vi "RVHR - Get Sum File Info.vi"(6 "Local Data in":T1, 8 "error in (no error)":errorcluster, 11 ".sum filepath":path) -> (0 "error out":errorcluster, 4 "Local Data out":T1)   [LabVIEW 2024]
uses:
  Controls/RVHR - Local Data.ctl
  Controls/Test Cluster.ctl
  Controls/Excluded Information.ctl
  Controls/Language.ctl
  Controls/Device_Type.ctl
  <vilib>/Utility/miscctls.llb/LVRectTypeDef.ctl
  <vilib>/Utility/miscctls.llb/LVBoundsTypeDef.ctl
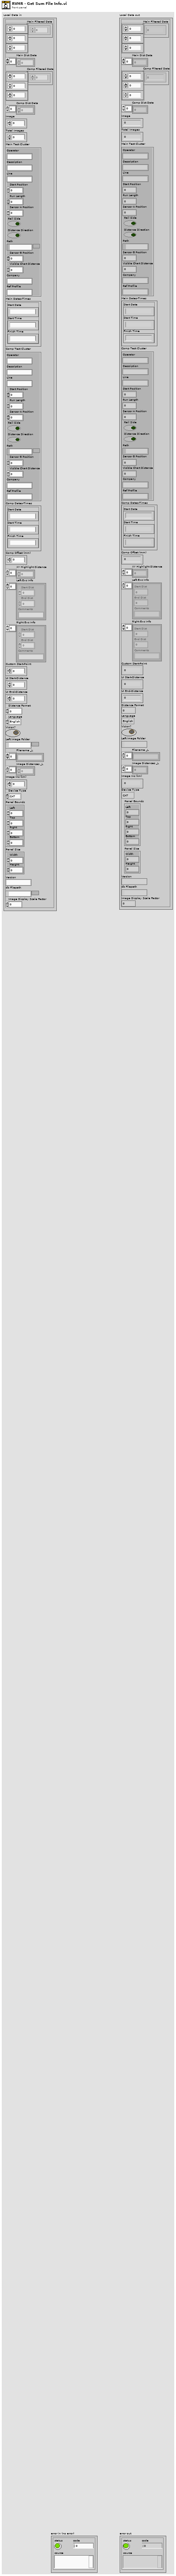
[diagram p1: front panel]
types:
  T1 = typedef "RVHR - Local Data.ctl" = cluster{"Main Filtered Data":dbl[][][], "Main Dist Data":dbl[], "Comp Filtered Data":dbl[][][], "Comp Dist Data":dbl[], "Image":u16, "Total Images":u16, "Main Test Cluster":T2, "Main Dates-Times":cluster{"Start Date":string, "Start Time":string, "Finish Time":string}, "Comp Test Cluster":T2, "Comp Dates-Times":cluster{"Start Date":string, "Start Time":string, "Finish Time":string}, "Comp Offset (mm)":i64, "XY Highlight Distance":dbl[], "Left Exc Info":T3[], "Right Exc Info":T3[], "Custom Start-Point":dbl, "UI Start-Distance":dbl, "UI End-Distance":dbl, "Distance Format":u8, "Language":T4, "Vision?":bool, "Left Image Folder":path, "Filename _L":string[], "Image Distances _L":dbl[], "Image Inc (km)":dbl, "Device Type":T5, "Panel Bounds":T6, "Panel Size":T7, "Version":string, "db Filepath":path, "Image Display Scale Factor":dbl}
  T2 = typedef "Test Cluster.ctl" = cluster{"Operator":string, "Description":string, "Line":string, "Start Position":dbl, "Run Length":dbl, "Sensor A Position":dbl, "Rail Side":bool, "Distance Direction":bool, "Path":path, "Sensor B Position":dbl, "Visible Chart Distance":dbl, "Company":string, "Ref Profile":string}
  T3 = typedef "Excluded Information.ctl" = cluster{"Start Dist":dbl, "End Dist":dbl, "Comments":string}
  T4 = typedef "Language.ctl" = enum16{"English", "Chinese", "German"}
  T5 = typedef "Device_Type.ctl" = enum16{"CAT", "Bi-CAT", "YRCA", "RCA", "RV-HR", "TV-HR"}
  T6 = typedef "LVRectTypeDef.ctl" = cluster{"Left":i16, "Top":i16, "Right":i16, "Bottom":i16}
  T7 = typedef "LVBoundsTypeDef.ctl" = cluster{"Width":u32, "Height":u32}
  T8 = cluster{"Start Date":string, "Start Time":string, "Finish Time":string}
  T9 = typedef "SUM Cluster.ctl" = cluster{"Test Cluster":T2, "Settings Cluster":T10, "End Distance":dbl, "Current Pos":dbl, "Start Pos":dbl, "Device_Type":T5, "Version":string}
  T10 = typedef "Settings Cluster.ctl" = cluster{"Sensor A Calibration":dbl, "Integrator Time":dbl, "Encoder Spacing":dbl, "Encoder Threshold":dbl, "Sampling Distance":T11, "Swap Direction?":bool, "Min Walking Speed":dbl, "Max Walking Speed":dbl, "Distance Format":T12, "Sensor B Calibration":dbl, "Tacho Pulses/Rev":dbl, "Wheel Diameter":dbl, "Max Short Roughness":dbl, "Max Long Roughness":dbl, "Measuring Interval":dbl, "Measuring Length":dbl, "Wavelengths":dbl[], "Device Resolution":T13, "Detect Change in Direction?":bool, "Save Images?":bool, "Image Frequency":T11, "Save Video?":bool, "Image Offset":dbl, "Start Position at 0m?":bool, "Live Corrug Est.?":bool, "Wavelength Corrug":u8, "Distance Corrug":u8, "Update Corrug":u8}
  T11 = typedef "Sampling DIstance.ctl" = u16
  T12 = typedef "Distance Units.ctl" = u16
  T13 = typedef "Device_Resolution.ctl" = u16
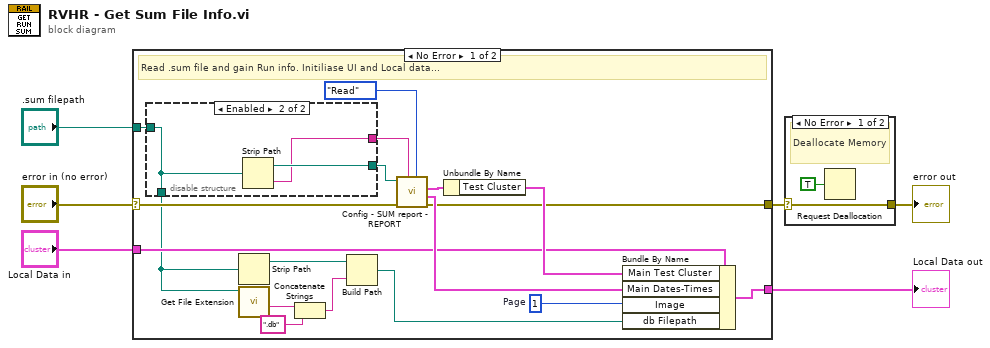
[diagram p0: block diagram]
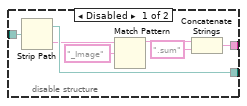
[diagram p3: hidden frame]
diagram:
  n1 = case shown="No Error" "error in (no error)" {
    selector: "error in (no error)" -> [w14 w36]
    tunnel: [w13 w36] -> w2
    tunnel: ".sum filepath" -> [w24 _]
    tunnel: [w21 w35] -> w5
    tunnel: "Local Data in" -> [w15 w35]
    frame No Error {
      w23 = u8 1  # Page
      # "Read .sum file and gain Run info. Initiliase UI and Local data..."
      n2 = disable-structure shown="Enabled" {
        disable-tunnel: w24 -> [w31 w32]
        disable-tunnel: [w30 w33] -> w20
        disable-tunnel: [w27 w34] -> w19
        disable-tunnel: [_ w32] -> w7
        frame Disabled {
          n3 = Strip Path(path=w31) -> (stripped path=w27:path, name=w26:string)
          n4 = Match Pattern(string=w26, regular expression="_Image") -> (before substring=w28:string)  [unwired: 1 in, 3 out]
          n5 = Concatenate Strings(w28, ".sum" ("string")) -> (w30:string)
        }
        frame Enabled {
          n6 = Strip Path(path=w32) -> (stripped path=w34:path, name=w33:string)
        }
      }
      n7 = Strip Path(path=w7) -> (stripped path=w12:path)  [unwired: 1 out]
      n8 = call <vilib>:"Get File Extension.vi"("file"=w7) -> ("filename without extension"=w11:string)  [unwired: 6 in, 4 out]
      n9 = Concatenate Strings(w11, ".db" ("string")) -> (w9:string)
      n10 = Build Path(base path=w12, name or relative path=w9) -> (appended path=w8:path)
      n11 = call "Config - SUM report - REPORT.vi"(".ini Controller"=enum16{"Read", "Write"}."Read", ".ini filename"=w20, "error in (no error)"=w14, "Directory Path"=w19) -> ("error out"=w13:errorcluster, "Dates-Times"=w22:T8, "Cluster out"=w17:T9)  [unwired: 5 in]
      n12 = Unbundle By Name(w17) -> ("Test Cluster"=w16:T2)
      n13 = Bundle By Name(cluster=w15, "Main Test Cluster"=w16, "Main Dates-Times"=w22, "Image"=w23, "db Filepath"=w8) -> (w21:T1)
    }
    frame Error {
    }
  }
  "Local Data out" <- w5
  n14 = case shown="No Error" w2 {
    selector: w2 -> [w37 w39]
    tunnel: [w37 w39] -> w1
    frame No Error {
      # "Deallocate Memory"
      n15 = Request Deallocation(TRUE ("flag")) -> ()
    }
    frame Error {
    }
  }
  "error out" <- w1
